vi "Bin Logging Message Loop.vi"(8 "error in (no error)":errorcluster, 10 "Data Queue":refnum<queue>, 11 "Message Queues":T1) -> (0 "error out":errorcluster)   [LabVIEW 2017, in "Logging.lvlib"]
uses:
  Logging.lvlib
  support/Message Queue/All Message Queues.ctl
  support/Message Queue/Message Cluster.ctl
  Logging Configuration.ctl
  Logging State.ctl
  support/Message Queue/Enqueue Message (Single).vi
  <vilib>/Utility/error.llb/Error Cluster From Error Code.vi
  <vilib>/ErrorRing/Error Ring.xnode
  support/Message Queue/Message Queue.lvlib
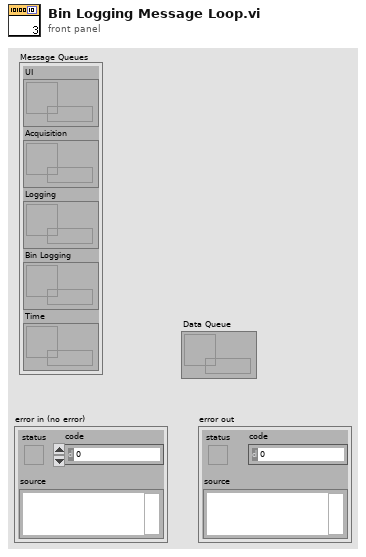
[diagram p1: front panel]
types:
  T1 = typedef "Message Queue.lvlib/All Message Queues.ctl" = cluster{"UI":refnum<queue>, "Acquisition":refnum<queue>, "Logging":refnum<queue>, "Bin Logging":refnum<queue>, "Time":refnum<queue>}
  T2 = typedef "Logging.lvlib/Logging Configuration.ctl" = cluster{"Log File Base Path":path, "TDMS File Reference":refnum<k34>, "Log File Offsite Path":path, "Offsite storage?":bool, "Project code":string, "Max writing time to a file [min]":dbl, "Bin File Reference":refnum<file>}
  T3 = enum16{"open", "replace", "create", "open or create", "replace or create", "replace or create with confirmation"}
  T4 = typedef "Logging.lvlib/Logging State.ctl" = enum16{"Idle", "Logging"}
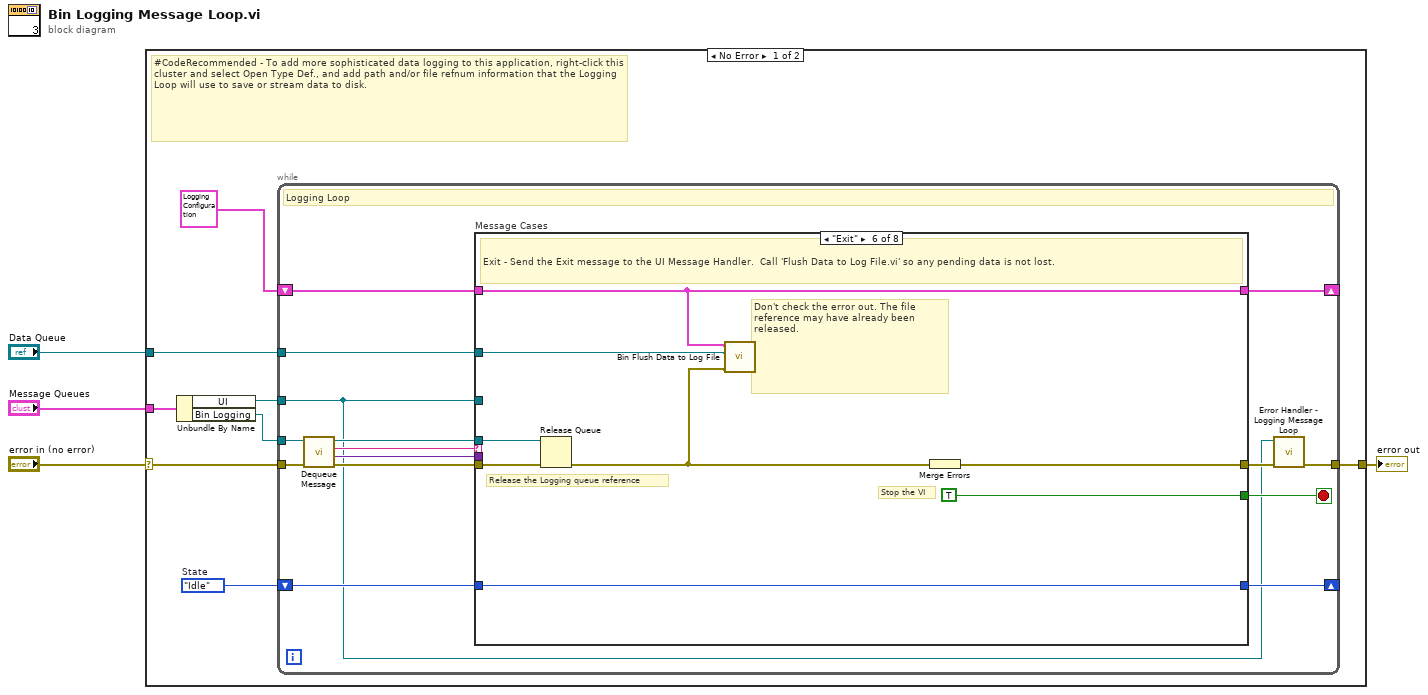
[diagram p0: block diagram]
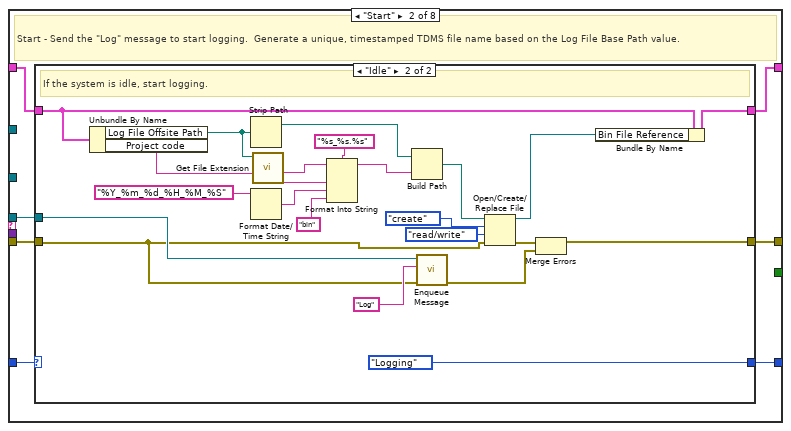
[diagram p3: hidden frame]
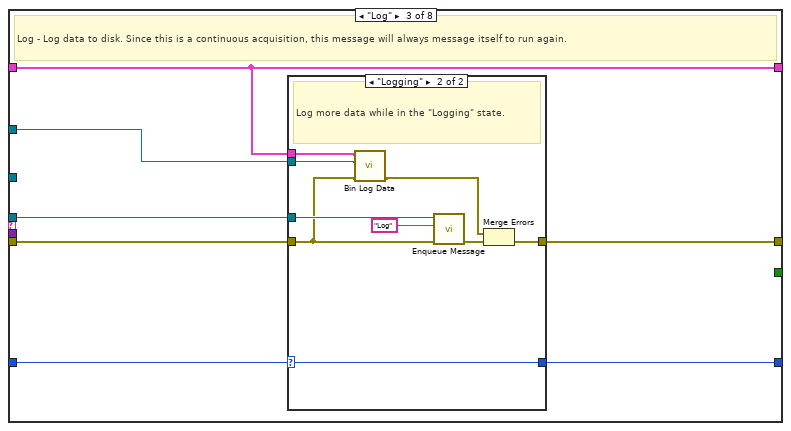
[diagram p5: hidden frame]
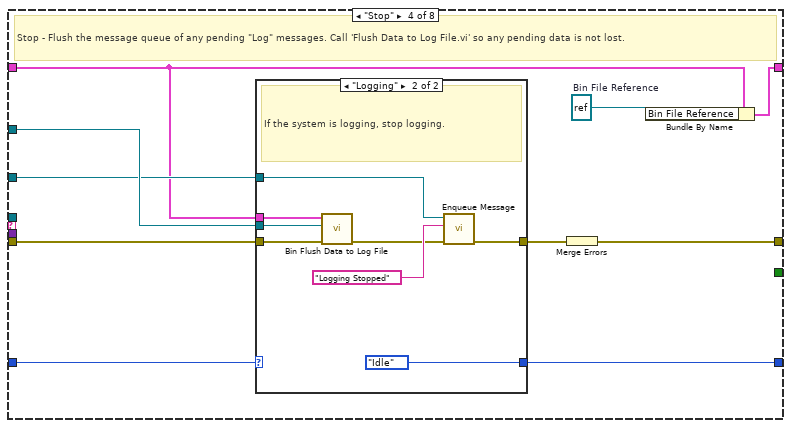
[diagram p7: hidden frame]
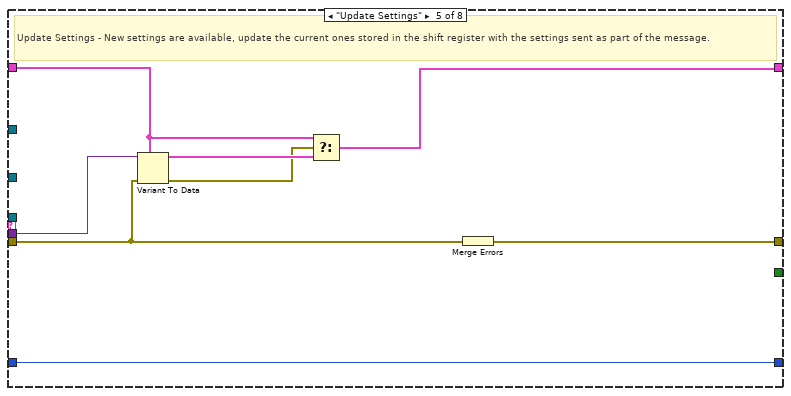
[diagram p9: hidden frame]
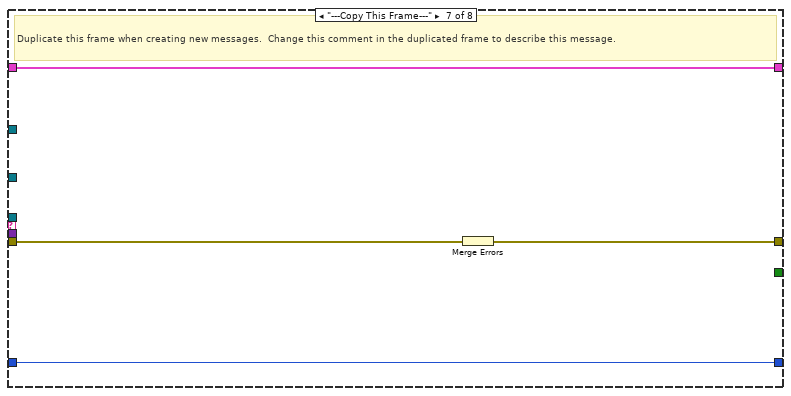
[diagram p10: hidden frame]
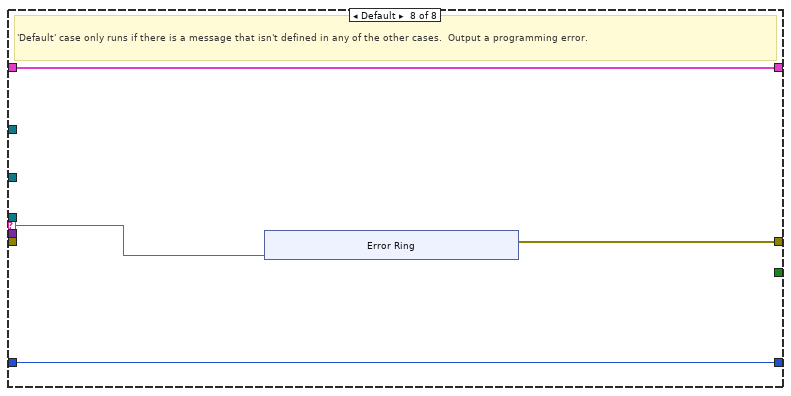
[diagram p11: hidden frame]
diagram:
  n1 = case shown="No Error" "error in (no error)" {
    selector: "error in (no error)" -> [w9 w132]
    tunnel: "Message Queues" -> [w12 _]
    tunnel: [w11 w132] -> w3
    tunnel: "Data Queue" -> [w8 _]
    frame No Error {
      w6 = Logging_State."Idle"  # State
      # "#CodeRecommended - To add more sophisticated data logging to this application, right-click this cluster and select Open Type Def., and add path and/or file refnum information that the Logging Loop will use to save or stream data to disk."
      n2 = Unbundle By Name(w12) -> ("UI"=w7:refnum<queue>, "Bin Logging"=w5:refnum<queue>)
      n3 = while {
        shift-right: [w26] -> _
        shift-left: T2 {"Log File Base Path"=path "", "TDMS File Reference"=refnum, "Log File Offsite Path"=path "", "Offsite storage?"=FALSE, "Project code"="", "Max writing time to a file [min]"=0.0, "Bin File Reference"=refnum} ("Logging Configuration") -> [w27]
        tunnel: w7 -> [w14]
        tunnel: w8 -> [w19]
        shift-right: [w17] -> _
        shift-left: w6 -> [w18]
        tunnel: w9 -> [w24]
        tunnel: [w16] -> w11
        tunnel: w5 -> [w13]
        stop <- w25 stop-if-true
        # "Logging Loop"
        n4 = call "Dequeue Message.vi"("error in (no error)"=w24, "Message Queue"=w13) -> ("error out"=w23:errorcluster, "Message Data"=w21:variant, "Message"=w22:string, "dup Message Queue"=w20:refnum<queue>)  [unwired: 6 in]
        n5 = case "Message Cases" shown="\"Exit\"" w22 {
          selector: w22 -> [_ _ _ _ _ _ _ w121]
          tunnel: w20 -> [_ w36 w68 _ _ w113 _ _]
          tunnel: w23 -> [w29 w35 w66 w87 w102 w114 w120 _]
          tunnel: [w29 w37 w69 w90 w108 w115 w118 w122] -> w15
          tunnel: w27 -> [w30 w34 w65 w82 w106 w111 w119 w124]
          tunnel: [w30 w33 w65 w81 w103 w111 w119 w124] -> w26
          tunnel: [_ _ _ _ _ TRUE _ _] -> w25
          tunnel: w21 -> [_ _ _ _ w107 _ _ _]
          tunnel: w14 -> [_ _ _ w84 _ _ _ _]
          tunnel: w19 -> [_ _ w67 w88 _ w109 _ _]
          tunnel: w18 -> [w28 w32 w64 w86 w101 w112 w117 w123]
          tunnel: [w28 w31 w63 w85 w101 w112 w117 w123] -> w17
          frame "Initialize" {
            # "Initialize - gets called when first launched. Currently a no-op."
          }
          frame "Start" {
            # "Start - Send the \"Log\" message to start logging.  Generate a unique, timestamped TDMS file name based on the Log File Base Path value."
            n6 = case shown="\"Idle\"" w32 {
              selector: w32 -> [w39 _]
              tunnel: [w38 w48] -> w37
              tunnel: w36 -> [_ w49]
              tunnel: w35 -> [w38 w42]
              tunnel: w34 -> [w40 w50]
              tunnel: [w40 w52] -> w33
              tunnel: [w39 Logging_State."Logging" ("State")] -> w31
              frame "Logging" {
                # "The system is already logging. Ignore the \"Start\" message."
              }
              frame "Idle" {
                # "If the system is idle, start logging."
                n7 = Unbundle By Name(w50) -> ("Log File Offsite Path"=w61:path, "Project code"=w47:string)
                n8 = Strip Path(path=w61) -> (stripped path=w58:path)  [unwired: 1 out]
                n9 = Format Date/Time String(time format string (%c)="%Y_%m_%d_%H_%M_%S") -> (date/time string=w56:string)  [unwired: 2 in]
                n10 = call <vilib>:"Get File Extension.vi"("file"=w61) -> ("filename without extension"=w59:string)  [unwired: 6 in, 4 out]
                n11 = Format Into String(format string="%s_%s.%s", initial string=w59, w47, w56, "bin" ("input 3")) -> (resulting string=w54:string)  [unwired: 1 in, 1 out]
                n12 = Build Path(base path=w58, name or relative path=w54) -> (appended path=w45:path)
                n13 = call-poly "Enqueue Message.vi"("error in (no error)"=w42, "Message"="Log", "Message Queue"=w49) -> ("error out"=w53:errorcluster)  [unwired: 7 in, 1 out]
                n14 = Open/Create/Replace File(file path (use dialog)=w45, error in=w42, operation (0:open)=T3."create", access (0:read/write)=enum16{"read/write", "read-only", "write-only"}."read/write") -> (refnum out=w41:refnum<file>, error out=w46:errorcluster)  [unwired: 2 in, 1 out]
                n15 = Merge Errors(w46, w53) -> (w48:errorcluster)
                n16 = Bundle By Name(cluster=w50, "Bin File Reference"=w41) -> (w52:T2)
              }
            }
          }
          frame "Log" {
            # "Log - Log data to disk. Since this is a continuous acquisition, this message will always message itself to run again."
            n17 = case shown="\"Logging\"" w64 {
              selector: w64 -> [w71 w76]
              tunnel: [w70 w80] -> w69
              tunnel: w68 -> [_ w78]
              tunnel: w67 -> [_ w74]
              tunnel: w66 -> [w70 w73]
              tunnel: w65 -> [_ w75]
              tunnel: [w71 w76] -> w63
              frame "Idle" {
                # "Ignore \"Log\" messages when the logging is idle."
              }
              frame "Logging" {
                # "Log more data while in the \"Logging\" state."
                n18 = call "Bin Log Data.vi"("error in (no error)"=w73, "Data Queue"=w74, "Logging Configuration"=w75) -> ("error out"=w72:errorcluster)  [unwired: 8 in]
                n19 = call-poly "Enqueue Message.vi"("error in (no error)"=w73, "Message"="Log", "Message Queue"=w78) -> ("error out"=w79:errorcluster)  [unwired: 7 in, 1 out]
                n20 = Merge Errors(w72, w79) -> (w80:errorcluster)
              }
            }
          }
          frame "Stop" {
            w83 = refnum<file> refnum  # Bin File Reference
            # "Stop - Flush the message queue of any pending \"Log\" messages. Call 'Flush Data to Log File.vi' so any pending data is not lost."
            n21 = case shown="\"Logging\"" w86 {
              selector: w86 -> [w91 _]
              tunnel: [w92 w99] -> w89
              tunnel: w88 -> [_ w95]
              tunnel: w82 -> [_ w96]
              tunnel: w87 -> [w92 w94]
              tunnel: [w91 Logging_State."Idle" ("State")] -> w85
              tunnel: w84 -> [_ w98]
              frame "Idle" {
                # "The system is already idle. Ignore the \"Stop\" message."
              }
              frame "Logging" {
                # "If the system is logging, stop logging."
                n22 = call "Bin Flush Data to Log File.vi"("error in (no error)"=w94, "Data Queue"=w95, "Logging Configuration"=w96) -> ("error out"=w93:errorcluster)  [unwired: 8 in]
                n23 = call-poly "Enqueue Message.vi"("error in (no error)"=w93, "Message"="Logging Stopped", "Message Queue"=w98) -> ("error out"=w99:errorcluster)  [unwired: 7 in, 1 out]
              }
            }
            n24 = Merge Errors(w89) -> (w90:errorcluster)
            n25 = Bundle By Name(cluster=w82, "Bin File Reference"=w83) -> (w81:T2)
          }
          frame "Update Settings" {
            # "Update Settings - New settings are available, update the current ones stored in the shift register with the settings sent as part of the message."
            n26 = Variant To Data(error in=w102, type=w106, Variant=w107) -> (data=w105:T2, error out=w104:errorcluster)
            n27 = Select(t=w106, s=w104, f=w105) -> (s? t:f=w103:T2)
            n28 = Merge Errors(w102) -> (w108:errorcluster)
          }
          frame "Exit" {
            # "Don't check the error out. The file reference may have already been released."
            # "Release the Logging queue reference"
            # "Stop the VI"
            # "Exit - Send the Exit message to the UI Message Handler.  Call 'Flush Data to Log File.vi' so any pending data is not lost."
            n29 = Release Queue(queue=w113, error in (no error)=w114) -> (error out=w110:errorcluster)  [unwired: 1 in, 2 out]
            n30 = call "Bin Flush Data to Log File.vi"("error in (no error)"=w110, "Data Queue"=w109, "Logging Configuration"=w111) -> ()  [unwired: 8 in, 1 out]
            n31 = Merge Errors(w110) -> (w115:errorcluster)
          }
          frame "---Copy This Frame---" {
            # "Duplicate this frame when creating new messages.  Change this comment in the duplicated frame to describe this message."
            n32 = Merge Errors(w120) -> (w118:errorcluster)
          }
          frame Default {
            # "'Default' case only runs if there is a message that isn't defined in any of the other cases.  Output a programming error."
            n33 = xnode "Error Ring"("parameter 0"=w121) -> ("error out"=w122:errorcluster)
          }
        }
        n34 = call "Error Handler - Logging Message Loop.vi"("error in (no error)"=w15, "Message Queue"=w14) -> ("dup error in"=w16:errorcluster)  [unwired: 8 in, 1 out]
      }
    }
    frame Error {
    }
  }
  "error out" <- w3
